vi "NML EventCounter.vi"() -> ()   [LabVIEW 2021]
doc: "I. Description:\nThis example demonstrates how to count digital events on a Counter Input Channel. The Initial Count, Count Direction, and Edge are all configurable. \n\nEdges are counted on the counter's default input terminal (see I/O Connections for more information), but could easily be modified to count edges on a PFI or RTSI line.\n\nII. Instructions for Running:\n1. Select the Physical Channel which corresponds to the counter you want to count edges on the DAQ device.\n2. Enter the Initial Count, Count Direction, and measurement Edge to specify how you want the counter to count. Additionally, you can change the input terminal where events are counted using the channel property node.\nNote: Use the Gen Dig Pulse Train-Continuous example to verify that you are counting correctly on the DAQ device.\n\nIII. Block Diagram Steps:\n1. Create a Counter Input channel to Count Events. The Edge parameter is used to determine if the counter will increment on rising or falling edges.\n2. Call the Start VI to arm the counter and begin counting. The counter will be preloaded with the Initial Count.\n3. The counter will be continually polled until the Stop button is pressed on the front panel.\n4. Call the Clear Task VI to clear the Task.\n5. Use the popup dialog box to display an error if any.\n\nIV. I/O Connections Overview:\nThe counter will count edges on the input terminal of the counter specified in the Physical Channel I/O control.\n\nIn this example the counter will count edges on the default input terminal on ctr0.\n\nFor more information on the default counter input and output terminals for your device, open the NI-DAQmx Help, and refer to Counter Signal Connections found under the Device Considerations book in the table of contents."
uses:
  <vilib>/Utility/error.llb/DialogType.ctl
  <vilib>/_DAQmxBase/Internals/DAQmxBase Create Channel (CI-Count Edges).vi
  <vilib>/_DAQmxBase/Internals/DAQmxBase Read (Counter U32 1Chan 1Samp).vi
panel:
  in  "Edge":i32(ring)=10171 items=["Rising"=10280, "Falling"=10171]
  in  "Count Direction":i32(ring)=10128 items=["Count Up"=10128, "Count Down"=10124, "Externally Controlled"=10326]
  in  "Initial Count":u32
  in  "Counter(s)":tag="Dev1/ctr0"
  out "Data":u32
  in  "stop":bool
  # "For instructions, select Help>>Show Context Help"
  # "Channel Parameters"
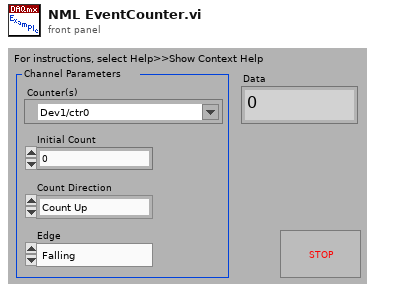
[diagram p1: front panel]
types:
  T1 = typedef "DialogType.ctl" = u16
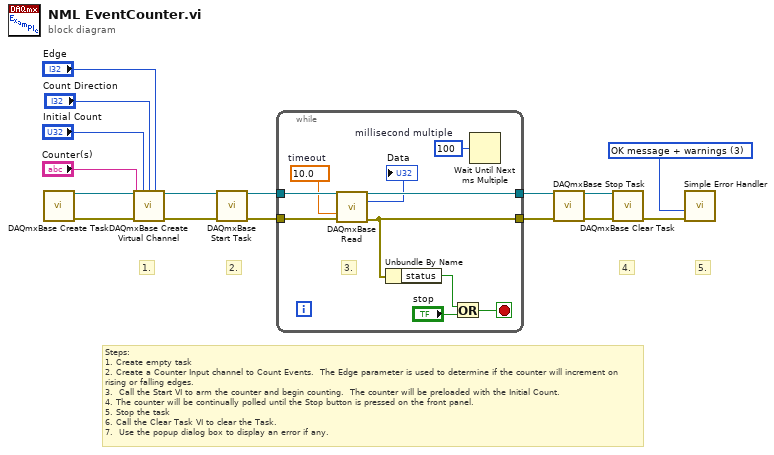
[diagram p0: block diagram]
diagram:
  w8 = T1 3 items=["no dialog", "OK message", "continue or stop message", "OK message + warnings", "continue/stop + warnings"] ("type of dialog (OK msg:1)")
  # "5."
  # "Steps: \n1. Create empty task\n2. Create a Counter Input channel to Count Events.  The Edge parameter is used to determine if the counter will increment on rising or falling edges.\n3.  Call the Start VI to arm the counter and begin counting.  The counter will be preloaded with the Initial Count.\n4. The counter will be continually polled until the Stop button is pressed on the front panel.\n5. Stop the task\n6. Call the Clear Task VI to clear the Task.\n7.  Use the popup dialog box to display an error if any."
  # "4."
  # "2."
  # "1."
  n1 = call <vilib>:"DAQmxBase Create Task.vi"() -> ("task out"=w5:refnum<k21>, "error out"=w6:errorcluster)  [unwired: 14 in]
  n2 = call-poly <vilib>:"DAQmxBase Create Virtual Channel.vi"("task in"=w5, "initial count"="Initial Count", "count direction"="Count Direction", "edge"="Edge", "counter"="Counter(s)", "error in"=w6) -> ("task out"=w12:refnum<k21>, "error out"=w13:errorcluster)  [unwired: 8 in]
  n3 = call <vilib>:"DAQmxBase Start Task.vi"("task/channels in"=w12, "error in"=w13) -> ("task out"=w14:refnum<k21>, "error out"=w16:errorcluster)  [unwired: 12 in]
  n4 = while {
    tunnel: w16 -> [w26]
    tunnel: [w22] -> w3
    tunnel: w14 -> [w21]
    tunnel: [w20] -> w4
    stop <- w25 stop-if-true
    w17 = u32 100  # millisecond multiple
    w18 = 10.0  # timeout
    # "3."
    n5 = call-poly <vilib>:"DAQmxBase Read.vi"("task/channels in"=w21, "timeout"=w18, "error in"=w26) -> ("task out"=w20:refnum<k21>, "data"=→"Data":u32, "error out"=w22:errorcluster)  [unwired: 10 in]
    n6 = Unbundle By Name(w22) -> ("status"=w23:bool)
    n7 = Or(x=w23, y="stop") -> (x .or. y?=w25:bool)
    n8 = Wait Until Next ms Multiple(millisecond multiple=w17) -> ()  [unwired: 1 out]
  }
  n9 = call <vilib>:"DAQmxBase Stop Task.vi"("task/channels in"=w4, "error in"=w3) -> ("task out"=w1:refnum<k21>, "error out"=w2:errorcluster)  [unwired: 12 in]
  n10 = call <vilib>:"DAQmxBase Clear Task.vi"("task in"=w1, "error in"=w2) -> ("error out"=w15:errorcluster)  [unwired: 13 in]
  n11 = call <vilib>:"Simple Error Handler.vi"("type of dialog (OK msg:1)"=w8, "error in (no error)"=w15) -> ()  [unwired: 3 in, 5 out]
